vi "AddFailure.vi"(7 "Time":dbl, 8 "error in (no error)":errorcluster, 9 "Failure":errorcluster, 10 "TestCase":refnum<class "TestCase.lvclass">, 11 "EventTestListener in":refnum<class "EventTestListener.lvclass">) -> (0 "error out":errorcluster, 3 "EventTestListener out":refnum<class "EventTestListener.lvclass">)   [LabVIEW 2019, in "TestExplorer.lvlib" / "EventTestListener.lvclass"]
doc: "A failure occurred."
uses:
  EventTestListener.lvclass
  TestCase/TestCase/TestCase.lvclass
  FailureEventData.ctl
  EventTestListener.lvclass/EventTestListener.ctl
  TestCase/Fact/Fact.lvclass
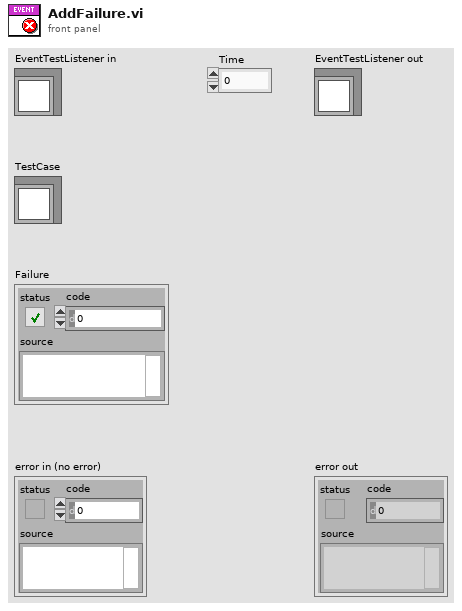
[diagram p1: front panel]
types:
  T1 = typedef "TestExplorer.lvlib/EventTestListener.lvclass/FailureEventData.ctl" = cluster{"TestCase":refnum<class "TestCase.lvclass">, "Failure":errorcluster, "Time":dbl}
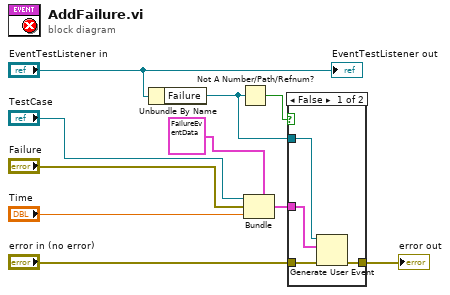
[diagram p0: block diagram]
diagram:
  n1 = Unbundle By Name("EventTestListener in") -> ("Failure"=w2:refnum<user-event>)
  n2 = Not A Number/Path/Refnum?(number/path/refnum=w2) -> (NaN/Path/Refnum?=w1:bool)
  n3 = Bundle(cluster=T1 {"TestCase"=refnum, "Failure"={"status"=TRUE, "code"=-8000, "source"="TestResultTest.lvlib:testPassed.vi<ERR>\nFailed asserting that actual size 0 matches expected size 1."}, "Time"=0.08753380000052857} ("FailureEventData"), "TestCase"="TestCase", "Failure"="Failure", "Time"="Time") -> (w3:T1)
  n4 = case shown="False" w1 {
    tunnel: "error in (no error)" -> [w14 w15]
    tunnel: [w13 w15] -> w9
    tunnel: w3 -> [w12 _]
    tunnel: w2 -> [w11 _]
    frame False {
      n5 = Generate User Event(user event=w11, event data cluster=w12, error in=w14) -> (error out=w13:errorcluster)  [unwired: 1 in, 1 out]
    }
    frame True {
    }
  }
  "error out" <- w9
  "EventTestListener out" <- "EventTestListener in"
